vi "Thermocouple.vi"() -> ()   [LabVIEW 2009]
uses:
  <vilib>/DAQmx/read.llb/DAQmx Read (Analog DBL 1Chan 1Samp).vi
  <vilib>/DAQmx/configure/timing.llb/DAQmx Timing (Sample Clock).vi
panel:
  in  "Sample Rate":dbl=1.0 format="%0.2f"
  out "Thermocouple Data":cluster{"Temperature Limit":dbl, "data":dbl}(graph)
  out "Limit Exceeded?":bool
  in  "Temperature Limit":dbl(slide)=30.0 scale=20.0..35.0
  in  "stop":bool
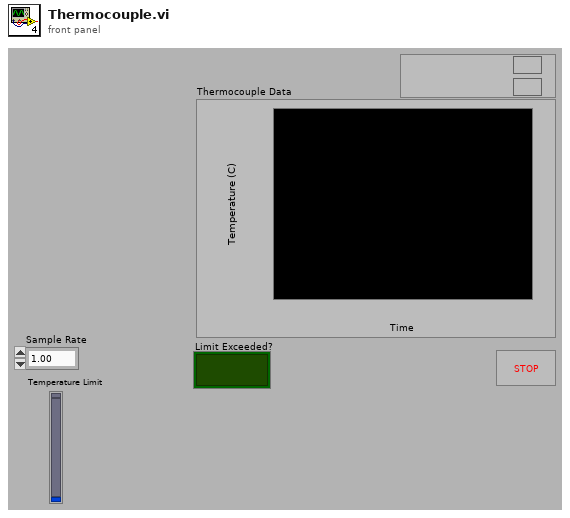
[diagram p1: front panel]
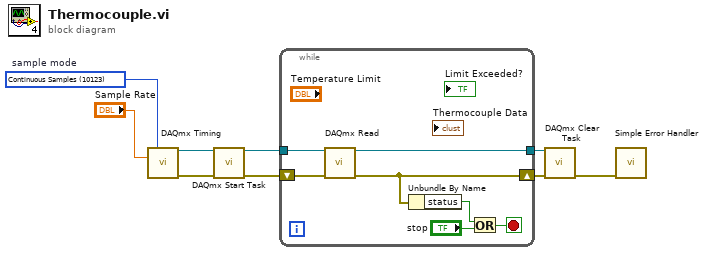
[diagram p0: block diagram]
diagram:
  w2 = 10123 items=["Finite Samples"=10178, "Continuous Samples"=10123, "Hardware Timed Single Point"=12522]  # sample mode
  n1 = call-poly <vilib>:"DAQmx Timing.vi"("sample mode"=w2, "rate"="Sample Rate") -> ("task out"=w4:refnum<k21>, "error out"=w3:errorcluster)  [unwired: 12 in]
  n2 = call <vilib>:"DAQmx Start Task.vi"("task/channels in"=w4, "error in"=w3) -> ("task out"=w7:refnum<k21>, "error out"=w6:errorcluster)  [unwired: 12 in]
  n3 = while {
    tunnel: [w16] -> w5
    tunnel: w7 -> [w14]
    shift-right: [w13] -> w9
    shift-left: w6 -> [w15]
    stop <- w12 stop-if-true
    n4 = call-poly <vilib>:"DAQmx Read.vi"("task/channels in"=w14, "error in"=w15) -> ("task out"=w16:refnum<k21>, "error out"=w13:errorcluster)  [unwired: 11 in, 1 out]
    n5 = Unbundle By Name "Unbundle By Name"(w13) -> ("status"=w11:bool)
    n6 = Or(x=w11, y="stop") -> (x .or. y?=w12:bool)
  }
  n7 = call <vilib>:"DAQmx Clear Task.vi"("task in"=w5, "error in"=w9) -> ("error out"=w8:errorcluster)  [unwired: 13 in]
  n8 = call <vilib>:"Simple Error Handler.vi"("error in (no error)"=w8) -> ()  [unwired: 4 in, 5 out]
